vi "CreateHandleWithoutLog.vi"   [LabVIEW 2015, in "MvCameraControl.lvlib"]
uses:
  MvCameraControl.lvlib
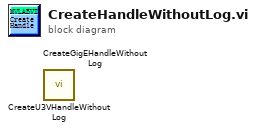
[diagram p0: block diagram]
diagram:
  n1 = call "CreateU3VHandleWithoutLog.vi"() -> ()  [unwired: 8 in, 3 out]
  n2 = call "CreateGigEHandleWithoutLog.vi"() -> ()  [unwired: 8 in, 3 out]
